vi "Actor Receive Decorator.vi"(11 "Dev Actor in":refnum<class "Dev Actor.lvclass">) -> (0 "error out":errorcluster, 2 "Msg":refnum<class "Msg Strategy.lvclass">, 3 "Dev Actor out":refnum<class "Dev Actor.lvclass">)   [LabVIEW 2021, in "Dev Actor.lvlib" / "Dev Actor.lvclass"]
uses:
  Dev Actor.lvclass
  src/LVCAM/LVCAM/Msg Strategy/Msg Strategy.lvclass
  Dev Actor.lvclass/Dev Actor.ctl
  src/LVCAM/LVCAM/Actor/Actor.lvclass
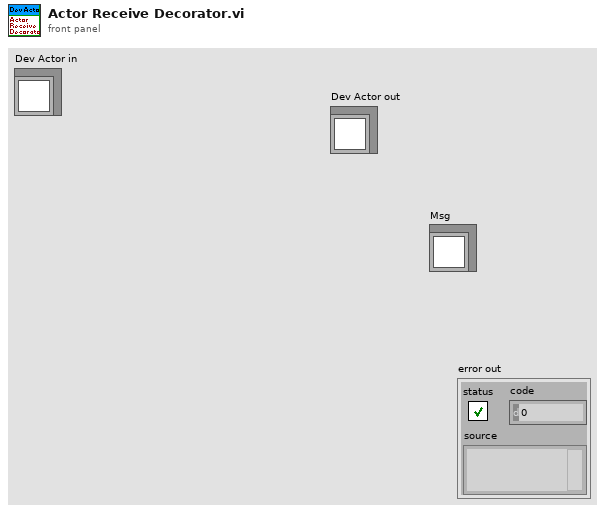
[diagram p1: front panel]
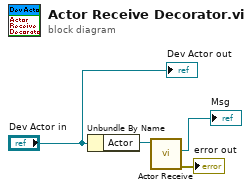
[diagram p0: block diagram]
diagram:
  n1 = Unbundle By Name("Dev Actor in") -> ("Actor"=w4:refnum<class "Actor.lvclass">)
  n2 = call-dynamic "Actor Receive.vi"("Actor in"=w4) -> ("error out"=→"error out":errorcluster, "Msg"=→"Msg":refnum<class "Msg Strategy.lvclass">)  [unwired: 8 in, 1 out]
  "Dev Actor out" <- "Dev Actor in"
